vi "Update State Name.vi"(8 "error in":errorcluster, 10 "State Name":string, 11 "ISeries UI Actor in":refnum<class "ISeries UI Actor.lvclass">) -> (0 "error out":errorcluster, 3 "ISeries UI Actor out":refnum<class "ISeries UI Actor.lvclass">)   [LabVIEW 2024, in "ISeries UI Actor.lvlib" / "ISeries UI Actor.lvclass"]
uses:
  ISeries UI Actor.lvclass
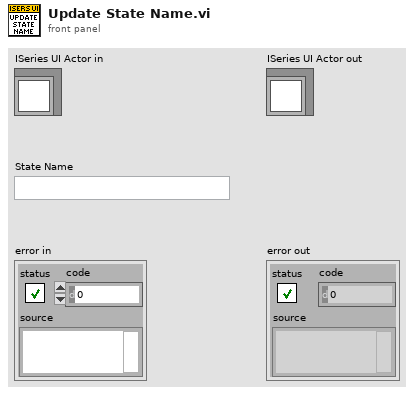
[diagram p1: front panel]
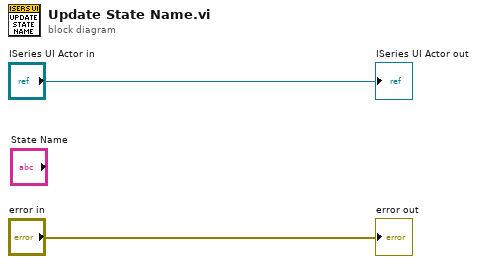
[diagram p0: block diagram]
diagram:
  "error out" <- "error in"
  "ISeries UI Actor out" <- "ISeries UI Actor in"
